vi "model_codeing.vi"() -> ()   [LabVIEW 2014]
uses:
  <vilib>/addons/Control Design/_Model Construction/Model Typedefs.llb/CD Transfer Function Model (MIMO).ctl
  <vilib>/addons/Control Design/_Model Construction/Model Typedefs.llb/CD General Elements.ctl
  <vilib>/addons/Control Design/_Model Construction/Model Typedefs.llb/CD Transfer Function Model (SISO).ctl
  <vilib>/addons/System Identification/Online Estimation.llb/SI Recursively Estimate ARX Model (SISO Waveform).vi
  <vilib>/addons/System Identification/Model Conversion.llb/SI Convert to Transfer Function Model of CDT.vi
  <vilib>/addons/Control Design/_Utility/Model Viewer.llb/Model Viewer SubVI/cd_Draw Transfer Function Equation (TF).vi
  <vilib>/addons/System Identification/Model Analysis.llb/SI Model Simulation (MISO Waveform).vi
  <vilib>/addons/System Identification/Model Analysis.llb/SI Model Prediction (MIMO Waveform).vi
  <vilib>/addons/System Identification/NI_SysID.lvlib
  <vilib>/gmath/NI_Gmath.lvlib
  <vilib>/Analysis/NI_AALPro.lvlib
  <vilib>/addons/Control Design/_Utility/NI_CD_Model Viewer.lvlib
  <vilib>/addons/Control Design/_Model Construction/NI_LinSys_Model Typedefs.lvlib
panel:
  out "Waveform Chart":dbl[](graph)
  out "appended array":dbl[](array[numeric])
  in  "?":T1(tab)
  out "STIMULUS":dynamicdata(graph) caption="Signals"
  out "RESPONSE":dynamicdata(graph) caption="Signals"
  out "RESPONSE VALIDATION":waveform(dbl)[](graph)
  out "XY Graph":T2(graph)
  in  "?":T3(tab)
  out "transfer function model":T4 {"transfer function(s)"."delay" format="%.4f"; "transfer function(s)"."Denominator" format="%#_3g"; "transfer function(s)"."Numerator" format="%#_3g"; "properties"."Sampling Time" format="%#.6p"; "properties"."Output Delays" format="%.4f"; "properties"."Input Delays" format="%.4f"}
  out "ARX Model Discret Transfer Function":picture
  in  "recursive method":enum16{"RLS", "KF", "NLMS", "LMS"}(ring)
  out "MSE":dbl format="%#.3g"
  in  "Fitting method":u16(ring) items=["Least Square", "Least Absolute Residual", "Bisquare"]
  out "Equation of fit":string
  in  "Display Precision":i32=3 min=0
  out "Fitted Data":dbl[](array[numeric]) format="%#.6g"
  out "X DATA":dbl[][](array[numeric])=[[0.01, 0.0], [1.0, 2.700000047683716], [2.0, 7.400000095367432], [3.0, 30.0], [4.0, 80.0], [5.0, 220.0]] format="%#.6g"
  out "Y DATA":dbl[][](array[numeric])=[[0.01, 0.0], [1.0, 2.700000047683716], [2.0, 7.400000095367432], [3.0, 30.0], [4.0, 80.0], [5.0, 220.0]] format="%#.6g"
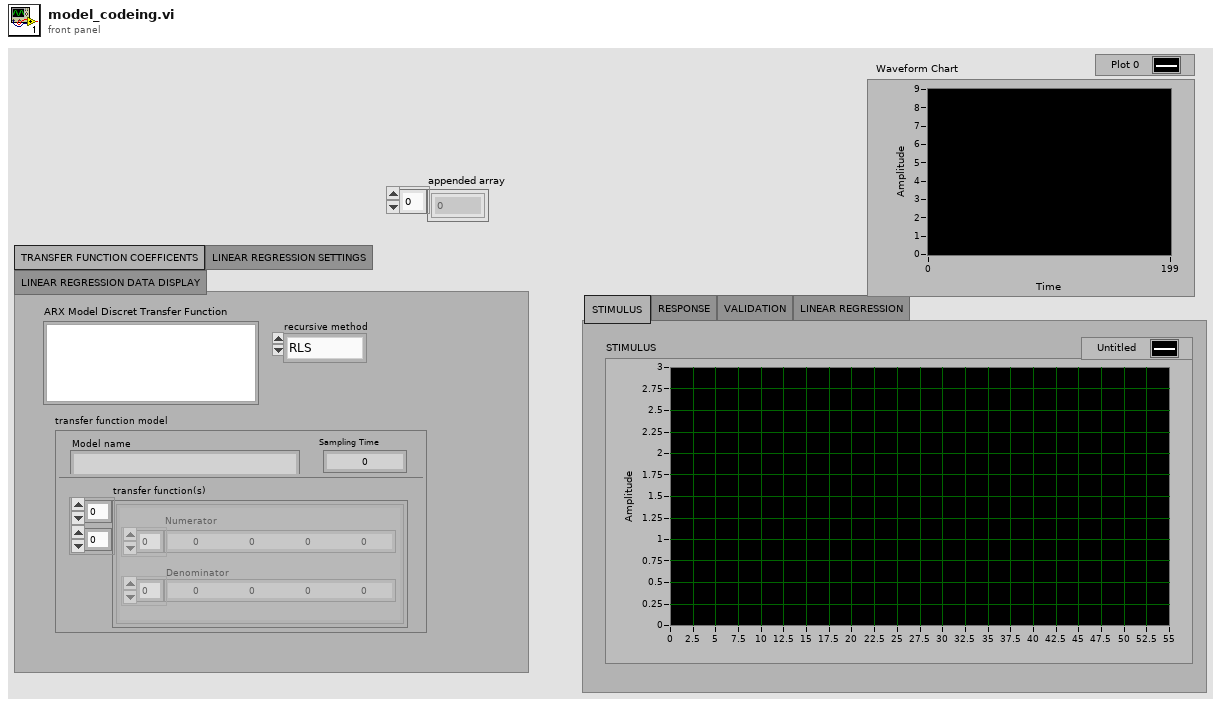
[diagram p1: front panel]
types:
  T1 = enum32{"STIMULUS ", "RESPONSE", "VALIDATION", "LINEAR REGRESSION"}
  T2 = cluster{"Data":dbl[], "Best Exponential Fit":dbl[]}[]
  T3 = enum32{"TRANSFER FUNCTION COEFFICENTS", "LINEAR REGRESSION SETTINGS", "LINEAR REGRESSION DATA DISPLAY"}
  T4 = typedef "NI_LinSys_Model Typedefs.lvlib/CD Transfer Function Model (MIMO).ctl" = cluster{"properties":T5, "transfer function(s)":T6[][]}
  T5 = typedef "NI_LinSys_Model Typedefs.lvlib/CD General Elements.ctl" = cluster{"Model name":string, "Input names":string[], "Output names":string[], "Input Delays":dbl[], "Output Delays":dbl[], "Sampling Time":dbl, "Notes":string}
  T6 = typedef "NI_LinSys_Model Typedefs.lvlib/CD Transfer Function Model (SISO).ctl" = cluster{"Numerator":dbl[], "Denominator":dbl[], "delay":dbl}
  T7 = enum16{"Linear", "Polynomial", "Exponential", "Power"}
  T8 = cluster{"A order":i32, "B order":i32, "delay":i32}
  T9 = typedef "NI_SysID.lvlib/si_generic model.ctl" = cluster{"attributes":cluster{"version":string, "model type":T10, "input names":string[], "output names":string[], "notes":string}, "coefficients":cluster{"A ":dbl[][][], "B":dbl[][][], "F":dbl[][][], "C":dbl[][][], "D":dbl[][][]}, "std deviations":cluster{"A ":dbl[][][], "B":dbl[][][], "F":dbl[][][], "C":dbl[][][], "D":dbl[][][]}, "coefficients covariance":dbl[][][], "noise variance":dbl[][], "fs":dbl, "system info":cluster{"number of inputs":i32, "number of outputs":i32, "A order":i32[][], "B order":i32[][], "F order":i32[][], "C order":i32[][], "D order":i32[][], "Delays":i32[][]}, "kalman gain":dbl[][], "initial state":dbl[], "trans func":cluster{"betas":dbl[], "alphas":dbl[]}[][], "zeros-poles":cluster{"zeros":cdb[], "poles":cdb[], "gain":dbl}[][], "std of trans func":cluster{"betas":dbl[], "alphas":dbl[]}[][], "std of zeros-poles":cluster{"zeros":cdb[], "poles":cdb[], "gain":dbl}[][], "trans func (noise)":cluster{"betas":dbl[], "alphas":dbl[]}[][], "std of trans func (noise)":cluster{"betas":dbl[], "alphas":dbl[]}[][], "zeros-poles (noise)":cluster{"zeros":cdb[], "poles":cdb[], "gain":dbl}[][], "std of zeros-poles (noise)":cluster{"zeros":cdb[], "poles":cdb[], "gain":dbl}[][], "Symbolic State Space Model":cluster{"Symbolic A":string[][], "Symbolic B":string[][], "Symbolic C":string[][], "Symbolic D":string[][], "Symbolic K":string[][], "Symbolic Initial State":string[]}, "delay":dbl[][], "variables":T11, "grey trans func spec":cluster{"orders of TF model":cluster{" num order":i32, "den order":i32}, "# of zeros/poles at origin":cluster{"zeros/poles":u16, "number ":i32}, "delay initial?":bool, "gain initial?":bool}}
  T10 = typedef "NI_SysID.lvlib/SI Model Type.ctl" = u16
  T11 = typedef "NI_SysID.lvlib/si_variables.ctl" = cluster{"name":string, "initial guess":dbl, "upper limit":dbl, "lower limit":dbl, "value":dbl}[]
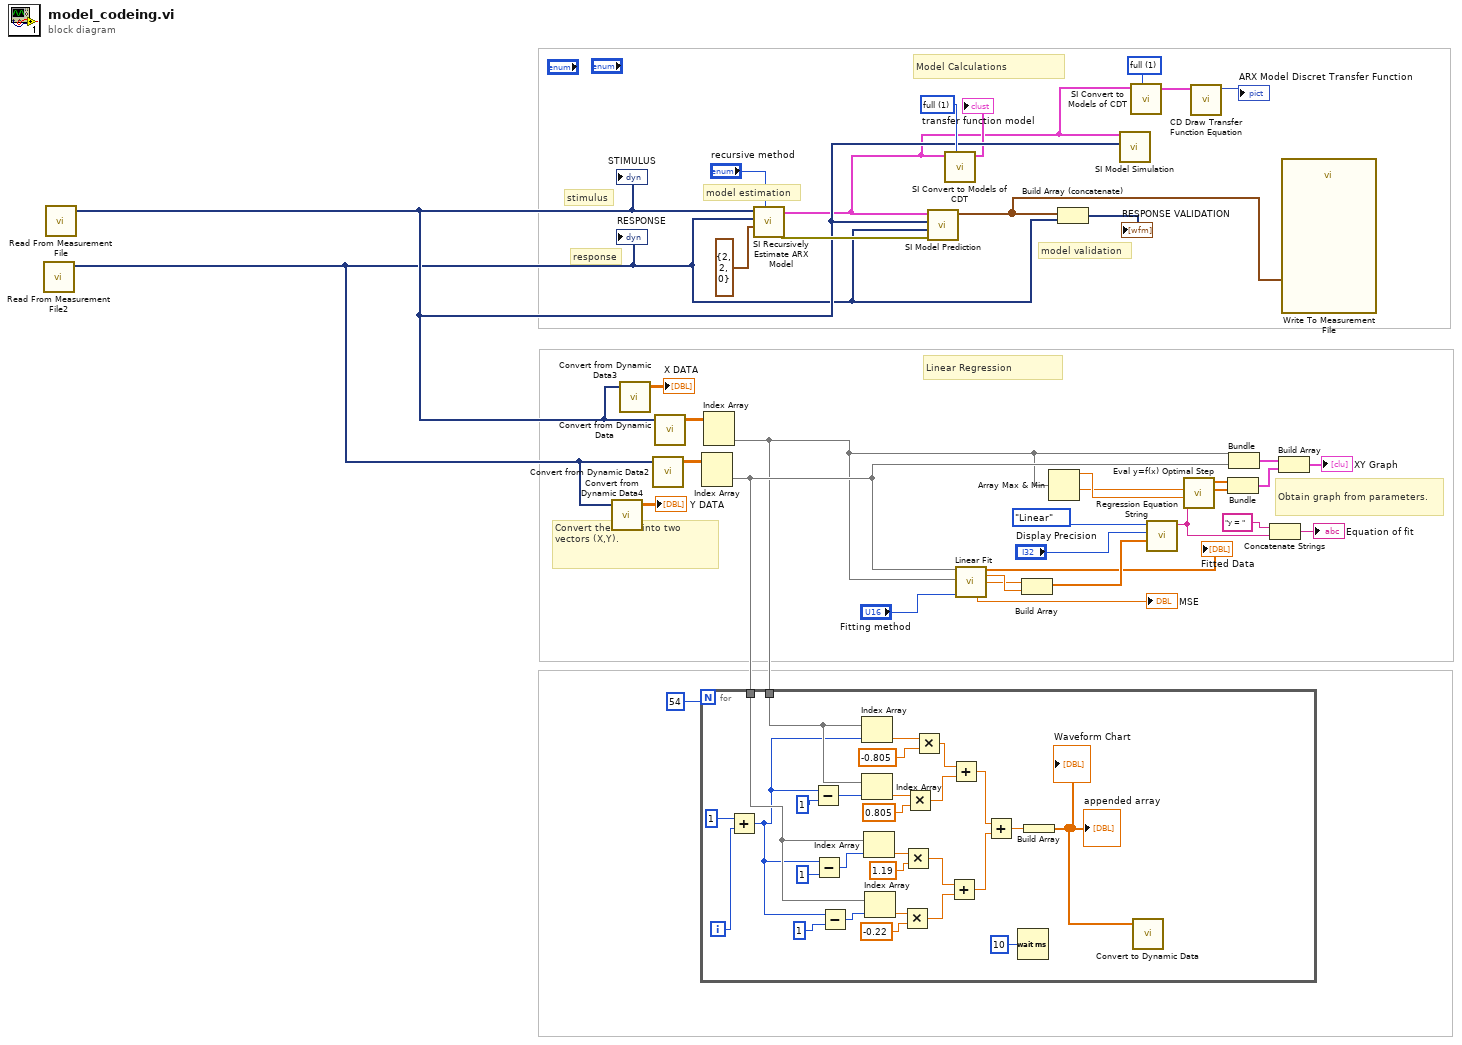
[diagram p0: block diagram]
diagram:
  w10 = u16 1 items=["minimum", "full"] ("realization type")
  w14 = u16 1 items=["minimum", "full"] ("realization type")
  # "Model Calculations"
  # "Linear Regression"
  # "model validation"
  # "model estimation"
  # "response"
  # "stimulus"
  # "Convert the table into two vectors (X,Y)."
  # "Obtain graph from parameters."
  n1 = call "Read From Measurement File2"() -> ("Signals"=w2:dynamicdata)  [unwired: 6 in, 5 out]
  "RESPONSE" <- w2
  n2 = call "Read From Measurement File"() -> ("Signals"=w13:dynamicdata)  [unwired: 6 in, 5 out]
  "STIMULUS" <- w13
  n3 = call "Convert from Dynamic Data4"("Dynamic Data Type"=w2) -> ("Array"=→"Y DATA":dbl[][])  [unwired: 3 in]
  n4 = call "Convert from Dynamic Data3"("Dynamic Data Type"=w13) -> ("Array"=→"X DATA":dbl[][])  [unwired: 3 in]
  n5 = call "Convert from Dynamic Data2"("Dynamic Data Type"=w2) -> ("Array"=w23:dbl[][])  [unwired: 3 in]
  n6 = call "Convert from Dynamic Data"("Dynamic Data Type"=w13) -> ("Array"=w18:dbl[][])  [unwired: 3 in]
  n7 = Index Array(array=w23) -> (element=w5:dbl[])  [unwired: 2 in]
  n8 = Index Array(array=w18) -> (element=w4:dbl[])  [unwired: 2 in]
  n9 = for {
    N: 54 -> [_]
    tunnel: w5 -> [w53]
    tunnel: w4 -> [w62]
    i -> [w66]
    n10 = Add(x=1, y=w66) -> (x+y=w52:i32)
    n11 = Subtract(x=w52, y=1) -> (x-y=w61:i32)
    n12 = Subtract(x=w52, y=1) -> (x-y=w55:i32)
    n13 = Subtract(x=w52, y=1) -> (x-y=w50:i32)
    n14 = Index Array(array=w62, index=w52) -> (element=w64:dbl)
    n15 = Index Array(array=w62, index=w61) -> (element=w59:dbl)
    n16 = Index Array(array=w53, index=w55) -> (element=w49:dbl)
    n17 = Index Array(array=w53, index=w50) -> (element=w47:dbl)
    n18 = Multiply(x=w47, y=-0.22) -> (x*y=w44:dbl)
    n19 = Multiply(x=w49, y=1.19) -> (x*y=w45:dbl)
    n20 = Multiply(x=w59, y=0.805) -> (x*y=w56:dbl)
    n21 = Multiply(x=w64, y=-0.805) -> (x*y=w57:dbl)
    n22 = Add(x=w45, y=w44) -> (x+y=w43:dbl)
    n23 = Add(x=w57, y=w56) -> (x+y=w42:dbl)
    n24 = Add(x=w42, y=w43) -> (x+y=w41:dbl)
    n25 = Wait (ms)(milliseconds to wait=u32 10) -> ()  [unwired: 1 out]
    n26 = Build Array(w41) -> (w40:dbl[])
    "appended array" <- w40
    "Waveform Chart" <- w40
    n27 = call "Convert to Dynamic Data"("Array"=w40) -> ()  [unwired: 3 in, 1 out]
  }
  n28 = call-poly <vilib>:"SI Recursively Estimate ARX Model.vi"("recursive method"="recursive method", "orders of ARX model"=T8 {"A order"=2, "B order"=2, "delay"=0}, "response signal"=w2, "stimulus signal"=w13) -> ("error out"=w20:errorcluster, "system model out"=w7:T9)  [unwired: 4 in, 2 out]
  n29 = call-poly <vilib>:"SI Model Prediction.vi"("error in (no error)"=w20, "response signals"=w2, "stimulus signals"=w13, "system model"=w7) -> ("predicted responses"=w1:waveform(dbl)[])  [unwired: 1 in, 6 out]
  n30 = call-poly <vilib>:"SI Convert to Models of CDT.vi"("realization type"=w14, "system model"=w7) -> ("transfer function model"=→"transfer function model":T4)  [unwired: 8 in, 1 out]
  n31 = call <vilib>:"Linear Fit.vi"("Y"=w5, "X"=w4, "method"="Fitting method") -> ("Best Linear Fit"=→"Fitted Data":dbl[], "slope"=w16:dbl, "intercept"=w15:dbl, "residue"=→"MSE":dbl)  [unwired: 8 in, 1 out]
  n32 = Build Array(w15, w16) -> (w35:dbl[])
  n33 = Array Max & Min(array=w4) -> (max value=w29:dbl, min value=w25:dbl)  [unwired: 2 out]
  n34 = Build Array (concatenate)(w2, w1) -> (→"RESPONSE VALIDATION":dynamicdata[])
  n35 = call-poly <vilib>:"SI Model Simulation.vi"("stimulus signals"=w13, "system model"=w7) -> ()  [unwired: 7 in, 3 out]
  n36 = call-poly <vilib>:"SI Convert to Models of CDT.vi"("realization type"=w10, "system model"=w7) -> ("transfer function model"=w8:T4)  [unwired: 2 in, 7 out]
  n37 = call "Regression Equation String.vi"("coefficients"=w35, "precision"="Display Precision", "fit type"=T7."Linear") -> ("Formula"=w26:string)  [unwired: 8 in]
  n38 = call <vilib>:"Eval y=f(x) Optimal Step.vi"("formula"=w26, "end"=w29, "start"=w25) -> ("Y Values"=w31:dbl[], "X Values"=w32:dbl[])  [unwired: 2 in, 2 out]
  n39 = call-poly <vilib>:"CD Draw Transfer Function Equation.vi"("Transfer Function Model"=w8) -> ("Equation"=→"ARX Model Discret Transfer Function":picture)  [unwired: 8 in, 2 out]
  n40 = Bundle("X Values"=w32, "Y Values"=w31) -> (w34:cluster{"X Values":dbl[], "Y Values":dbl[]})  [unwired: 1 in]
  n41 = Bundle("Array"=w4, "Array"=w5) -> (w36:cluster{"Array":dbl[], "Array":dbl[]})  [unwired: 1 in]
  n42 = Concatenate Strings("y = " ("string"), w26) -> (→"Equation of fit":string)
  n43 = Build Array(w36, w34) -> (→"XY Graph":cluster{"X Values":dbl[], "Y Values":dbl[]}[])
  n44 = call "Write To Measurement File"("Signals"=w1) -> ()  [unwired: 16 in, 3 out]
